vi "Read_Camera.vi"(7 "data type":u16(ring) items=["array", "spectrum"], 10 "Image Handle IN":u32 caption="Image Handle", 11 "input parameters":T1={"camera parameters"={"Camera Handle"=16842752, "Xdim"=1340, "Ydim"=400}, "error"={"status"=FALSE, "code"=0, "source"=""}, "Plot height [pixel]"=0.0, "Plot width [pixel]"=0.0}) -> (0 "array":dbl[][](array[numeric]), 1 "spectrum":dbl[](array[numeric]), 2 "Image Handle OUT":u32, 3 "output parameters":T1={"camera parameters"={"Camera Handle"=16842752, "Xdim"=1340, "Ydim"=400}, "error"={"status"=FALSE, "code"=0, "source"=""}, "Plot height [pixel]"=0.0, "Plot width [pixel]"=0.0}, 4 "exit program":bool)   [LabVIEW 2013]
uses:
  Instance           1 19Saved   Read_Camera .vi
panel:
  out "Count":dbl
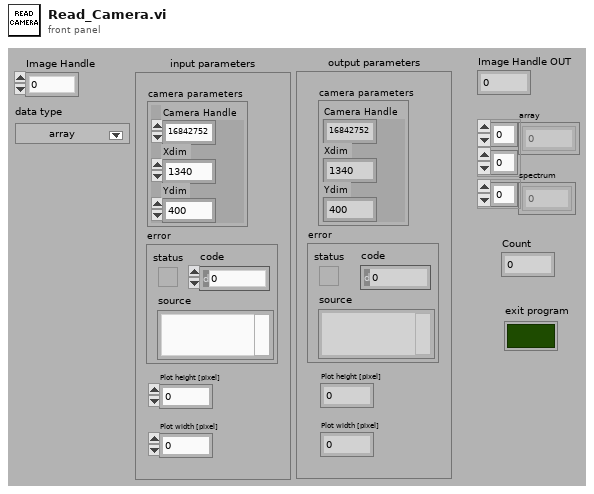
[diagram p1: front panel]
types:
  T1 = cluster{"camera parameters":cluster{"Camera Handle":u32, "Xdim":u32, "Ydim":u32}, "error":errorcluster, "Plot height [pixel]":dbl, "Plot width [pixel]":dbl}
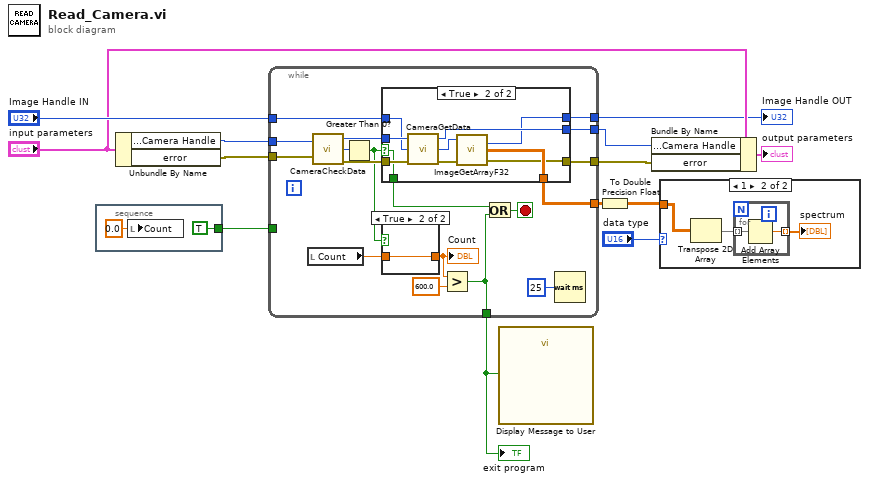
[diagram p0: block diagram]
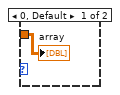
[diagram p2: hidden frame]
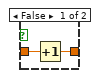
[diagram p3: hidden frame]
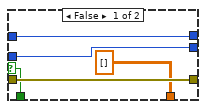
[diagram p4: hidden frame]
diagram:
  n1 = stacked-sequence {
    tunnel: [TRUE] -> w5
    frame #0 {
      n2 = local write "Count"(0.0 ("Count")) -> ()
    }
  }
  n3 = Unbundle By Name("input parameters") -> ("camera parameters.Camera Handle"=w9:u32, "error"=w10:errorcluster)
  n4 = while {
    tunnel: [w33] -> w7
    tunnel: [w32] -> w8
    tunnel: "Image Handle IN" -> [w28]
    tunnel: w9 -> [w27]
    tunnel: w10 -> [w26]
    tunnel: [w25] -> w6
    tunnel: [w18] -> w4
    tunnel: w5 -> [_]
    tunnel: [w17] -> w3
    stop <- w20 stop-if-true
    n5 = local read "Count"() -> (w23:dbl)
    n6 = call <userlib>:"CameraCheckData.vi"("Camera Handle"=w27, "error in"=w26) -> ("Camera Handle"=w29:u32, "Number Of Frames Available"=w30:i32, "error out"=w31:errorcluster)
    n7 = Greater Than 0?(x=w30) -> (x > 0?=w24:bool)
    n8 = case shown="True" w24 {
      selector: w24 -> [w39 w47]
      tunnel: w31 -> [w41 w51]
      tunnel: w29 -> [w40 w50]
      tunnel: [w40 w49] -> w32
      tunnel: [w41 w43] -> w33
      tunnel: [w39 w47] -> w19
      tunnel: [sgl[][] [] ("Array Float 32") w45] -> w17
      tunnel: w28 -> [w37 w44]
      tunnel: [w37 w42] -> w25
      frame False {
      }
      frame True {
        n9 = call <userlib>:"CameraGetData.vi"("error in"=w51, "Data Handle"=w44, "Camera Handle"=w50) -> ("error out"=w48:errorcluster, "Data Handle"=w46:u32, "Camera Handle"=w49:u32)
        n10 = call <userlib>:"ImageGetArrayF32.vi"("error in"=w48, "Image Handle"=w46) -> ("error out"=w43:errorcluster, "Array Float 32"=w45:sgl[][], "Image Handle"=w42:u32)  [unwired: 1 in]
      }
    }
    n11 = case shown="True" w24 {
      tunnel: [w35 w36] -> w22
      tunnel: w23 -> [w34 w36]
      frame False {
        n12 = Increment(x=w34) -> (x+1=w35:dbl)
      }
      frame True {
      }
    }
    "Count" <- w22
    n13 = Greater?(x=w22, y=600.0) -> (0:w18:bool)
    n14 = Or(x=w19, y=w18) -> (x .or. y?=w20:bool)
    n15 = Wait (ms)(milliseconds to wait=u32 25 ("Zu wartende ms")) -> ()  [unwired: 1 out]
  }
  "Image Handle OUT" <- w6
  "exit program" <- w4
  n16 = call "Display Message to User"("Enable"=w4) -> ()  [unwired: 9 in, 2 out]
  n17 = To Double Precision Float(number=w3) -> (double precision float=w2:dbl[][])
  n18 = Bundle By Name(cluster="input parameters", "camera parameters.Camera Handle"=w8, "error"=w7) -> (→"output parameters":T1)
  n19 = case shown="1" "data type" {
    tunnel: w2 -> [w52 w53]
    frame 0, Default {
      "array" <- w52
    }
    frame 1 {
      n20 = Transpose 2D Array(2D array=w53) -> (transposed array=w55:dbl[][])
      n21 = for {
        tunnel: w55 -> [w57] mode=indexing
        tunnel: [w56] -> w54 mode=indexing
        n22 = Add Array Elements(numeric array=w57) -> (sum=w56:dbl)
      }
      "spectrum" <- w54
    }
  }
